vi "QMH-SM Hybrid example program.vi"() -> ()   [LabVIEW 2010]
uses:
  States_2.ctl
panel:
  in  "Stop":bool
  in  "Start":bool
  out "Waveform Chart":dbl(graph)
  in  "Max Value":dbl=20.0
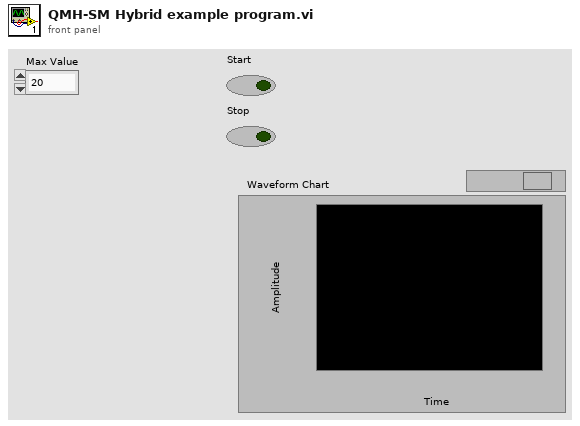
[diagram p1: front panel]
types:
  T1 = typedef "States_2.ctl" = enum16{"Stop", "Initialize", "Add to Plot", "Add More Data"}
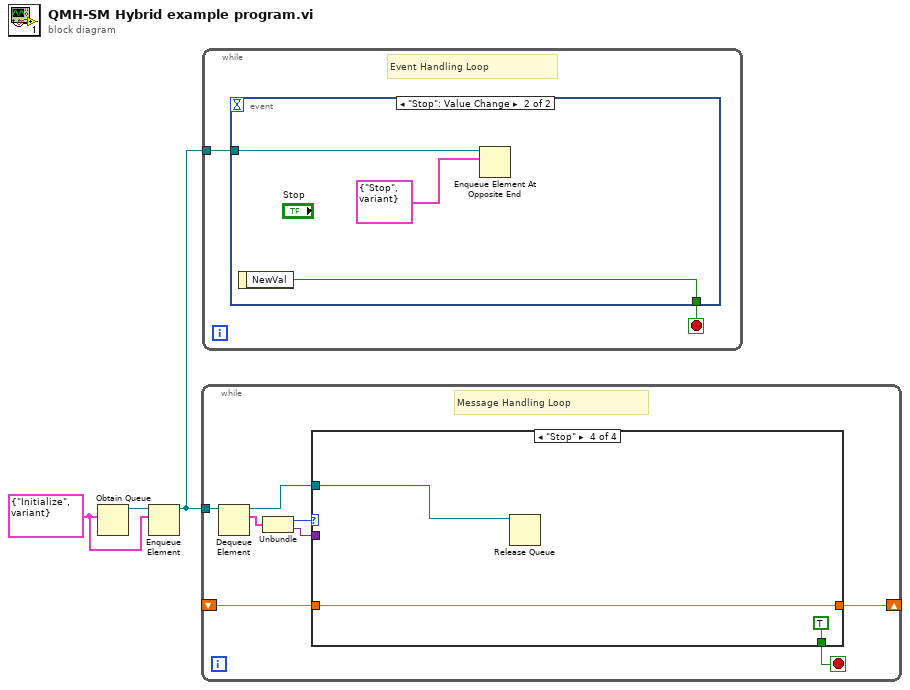
[diagram p0: block diagram]
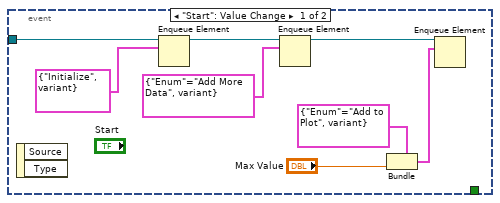
[diagram p2: hidden frame]
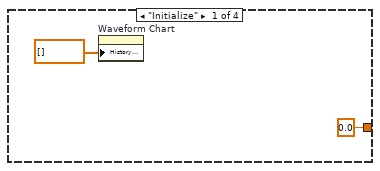
[diagram p3: hidden frame]
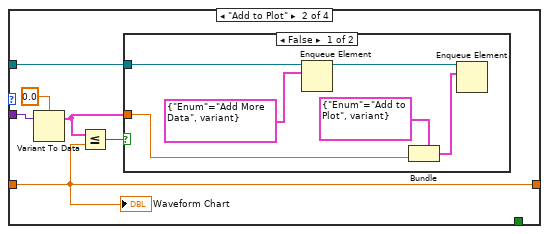
[diagram p4: hidden frame]
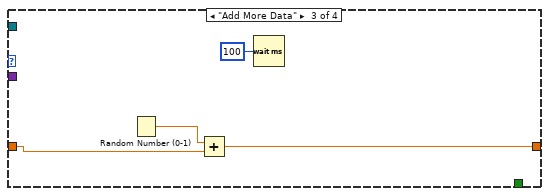
[diagram p6: hidden frame]
diagram:
  w1 = cluster{"Enum":T1, variant} {"Enum"=enum."Initialize", variant} ("element")
  n1 = Obtain Queue(element data type=w1) -> (queue out=w3:refnum<queue>)  [unwired: 4 in, 2 out]
  n2 = Enqueue Element(queue=w3, element=w1) -> (queue out=w2:refnum<queue>)  [unwired: 2 in, 2 out]
  n3 = while {
    tunnel: w2 -> [w11]
    shift-right: [w5] -> _
    shift-left: _ -> [w4]
    stop <- w8 stop-if-true
    # "Message Handling Loop"
    n4 = Dequeue Element(queue=w11) -> (queue out=w7:refnum<queue>, element=w10:cluster{"Enum":T1, variant})  [unwired: 2 in, 2 out]
    n5 = Unbundle(w10) -> ("Enum"=w6:T1, w9:variant)
    n6 = case shown="\"Stop\"" w6 {
      tunnel: w9 -> [_ w19 _ _]
      tunnel: [_ _ _ TRUE] -> w8
      tunnel: w7 -> [_ w14 _ w30]
      tunnel: [0.0 w17 w28 w31] -> w5
      tunnel: w4 -> [_ w17 w27 w31]
      frame "Initialize" {
        n7 = property on="Waveform Chart" class="WFChart (strict)"("History Data"=dbl[] []) -> ()  [unwired: 2 in, 2 out]
      }
      frame "Add to Plot" {
        n8 = Variant To Data(Variant=w19, type=0.0) -> (data=w15:cluster{})  [unwired: 1 in, 1 out]
        n9 = Less Or Equal?(x=w15, y=w17) -> (x <= y?=w16:bool)
        n10 = case shown="False" w16 {
          tunnel: w15 -> [w21 _]
          tunnel: w14 -> [w20 _]
          frame False {
            n11 = Enqueue Element(queue=w20, element=cluster{"Enum":T1, variant} {"Enum"=enum."Add More Data", variant}) -> (queue out=w24:refnum<queue>)  [unwired: 2 in, 2 out]
            n12 = Bundle(cluster=cluster{"Enum":T1, variant} {"Enum"=enum."Add to Plot", variant} ("element"), w21) -> (w25:cluster{"Enum":T1, variant})  [unwired: 1 in]
            n13 = Enqueue Element(queue=w24, element=w25) -> ()  [unwired: 2 in, 3 out]
          }
          frame True {
          }
        }
        "Waveform Chart" <- w17
      }
      frame "Add More Data" {
        n14 = Random Number (0-1)() -> (number: 0 to 1=w29:dbl)
        n15 = Add(x=w29, y=w27) -> (x+y=w28:dbl)
        n16 = Wait (ms)(milliseconds to wait=u32 100) -> ()  [unwired: 1 out]
      }
      frame "Stop" {
        n17 = Release Queue(queue=w30) -> ()  [unwired: 2 in, 3 out]
      }
    }
  }
  n18 = while {
    tunnel: w2 -> [w34]
    stop <- w33 stop-if-true
    # "Event Handling Loop"
    n19 = event shown="[1] \"Stop\": Value Change" {
      selector: _ -> [_ _]
      dyn-events: _ -> [_ _]
      timeout: _ -> [_ _]
      tunnel: w34 -> [w41 w43]
      tunnel: [_ w45] -> w33
      event "Start": Value Change {
        n20 = event-data() -> ()  [unwired: 1 in, 2 out]
        n21 = Enqueue Element(queue=w41, element=cluster{"Enum":T1, variant} {"Enum"=enum."Initialize", variant}) -> (queue out=w39:refnum<queue>)  [unwired: 2 in, 2 out]
        n22 = Enqueue Element(queue=w39, element=cluster{"Enum":T1, variant} {"Enum"=enum."Add More Data", variant}) -> (queue out=w38:refnum<queue>)  [unwired: 2 in, 2 out]
        n23 = Bundle(cluster=cluster{"Enum":T1, variant} {"Enum"=enum."Add to Plot", variant} ("element"), "Max Value") -> (w36:cluster{"Enum":T1, variant})  [unwired: 1 in]
        n24 = Enqueue Element(queue=w38, element=w36) -> ()  [unwired: 2 in, 3 out]
      }
      event "Stop": Value Change {
        n25 = event-data() -> ("NewVal"=w45:bool)  [unwired: 1 in]
        n26 = Enqueue Element At Opposite End(queue=w43, element=cluster{"Enum":T1, variant} {"Enum"=enum."Stop", variant}) -> ()  [unwired: 2 in, 3 out]
      }
    }
  }
